vi "NormalizeYAxis (SubVI).vi"(6 "negative?":bool, 10 "Yaxis":i32) -> (2 "NormalizedAxis":dbl)   [LabVIEW 2020]
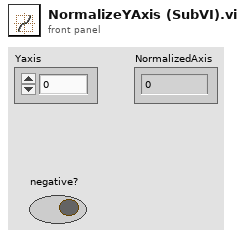
[diagram p1: front panel]
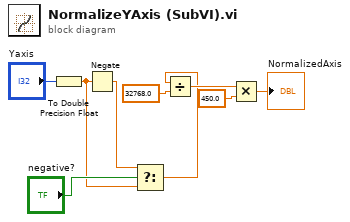
[diagram p0: block diagram]
diagram:
  n1 = To Double Precision Float(number="Yaxis") -> (double precision float=w2:dbl)
  n2 = Negate(x=w2) -> (-x=w3:dbl)
  n3 = Select(t=w3, s="negative?", f=w2) -> (s? t:f=w1:dbl)
  n4 = Divide(x=w1, y=32768.0) -> (x/y=w7:dbl)
  n5 = Multiply(x=w7, y=450.0) -> (x*y=→"NormalizedAxis":dbl)
